vi "PIDController_Calculate_PV.vi"(10 "PV":dbl, 11 "in PID_CONTROLLER":T1={"Kp"=0.0, "Ki"=0.0, "Kd"=0.0, "Period"=0.0, "Max_Integral"=0.0, "Min_Integral"=0.0, "Max_Input"=0.0, "Min_Input"=0.0, "Continuous"=FALSE, "PositionError"=0.0, "VelocityError"=0.0, "PrevError"=0.0, "Total_Integral"=0.0, "PositionTolerance"=0.0, "VelocityTolerance"=0.0, "SetPoint"=0.0, "Kf"=0.0, "Prev_Deriv"=0.0, "Prev_Deriv 2"=0.0, "DerivativeFilter"=FALSE, "Min_Output"=-9.99e+35, "Max_Output"=9.9e+35, "Prev_F_P"=0.0, "Prev_F_P_2"=0.0, "AntiWindupActive"=FALSE, "Measurement"=0.0, "IntegralZone"=9.9e+30} {"IntegralZone" format="%16_6e"; "Measurement" format="%16_6e"; "Prev_F_P_2" format="%16_6e"; "Prev_F_P" format="%16_6e"; "Max_Output" format="%16_6e"; "Min_Output" format="%16_6e"; "Prev_Deriv 2" format="%16_6e"; "Prev_Deriv" format="%16_6e"; "Kf" format="%16_6e"; "SetPoint" format="%16_6e"; "VelocityTolerance" format="%16_6e"; "PositionTolerance" format="%16_6e"; "Total_Integral" format="%16_6e"; "PrevError" format="%16_6e"; "VelocityError" format="%16_6e"; "PositionError" format="%16_6e"; "Min_Input" format="%16_6e"; "Max_Input" format="%16_6e"; "Min_Integral" format="%16_6e"; "Max_Integral" format="%16_6e"; "Period" format="%16_6e"; "Kd" format="%16_6e"; "Ki" format="%16_6e"; "Kp" format="%16_6e"}) -> (1 "ControlOutput":dbl, 3 "out PID_CONTROLLER":T1={"Kp"=0.0, "Ki"=0.0, "Kd"=0.0, "Period"=0.0, "Max_Integral"=0.0, "Min_Integral"=0.0, "Max_Input"=0.0, "Min_Input"=0.0, "Continuous"=FALSE, "PositionError"=0.0, "VelocityError"=0.0, "PrevError"=0.0, "Total_Integral"=0.0, "PositionTolerance"=0.0, "VelocityTolerance"=0.0, "SetPoint"=0.0, "Kf"=0.0, "Prev_Deriv"=0.0, "Prev_Deriv 2"=0.0, "DerivativeFilter"=FALSE, "Min_Output"=-9.99e+35, "Max_Output"=9.9e+35, "Prev_F_P"=0.0, "Prev_F_P_2"=0.0, "AntiWindupActive"=FALSE, "Measurement"=0.0, "IntegralZone"=9.9e+30} {"IntegralZone" format="%16_6e"; "Measurement" format="%16_6e"; "Prev_F_P_2" format="%16_6e"; "Prev_F_P" format="%16_6e"; "Max_Output" format="%16_6e"; "Min_Output" format="%16_6e"; "Prev_Deriv 2" format="%16_6e"; "Prev_Deriv" format="%16_6e"; "Kf" format="%16_6e"; "SetPoint" format="%16_6e"; "VelocityTolerance" format="%16_6e"; "PositionTolerance" format="%16_6e"; "Total_Integral" format="%16_6e"; "PrevError" format="%16_6e"; "VelocityError" format="%16_6e"; "PositionError" format="%16_6e"; "Min_Input" format="%16_6e"; "Max_Input" format="%16_6e"; "Min_Integral" format="%16_6e"; "Max_Integral" format="%16_6e"; "Period" format="%16_6e"; "Kd" format="%16_6e"; "Ki" format="%16_6e"; "Kp" format="%16_6e"})   [LabVIEW 2019, in "Trajectory_Library.lvlib"]
doc: "Returns the next output of the PID controller. The saved setpoint (SP) in the PID_Controller data structure is used.\n \nInputs:\n - PID_Controller -- PID_Controller data cluster\n - PV-measurement -- The current measurement of the process variable. (PV)\n\nOutputs:\n - PID_Controller -- Updated PID_Controller data cluster\n - CO-ControlOutput -- Controller output (CO)"
uses:
  Trajectory_Library.lvlib
  TypeDef/PID_CONTROLLER.ctl
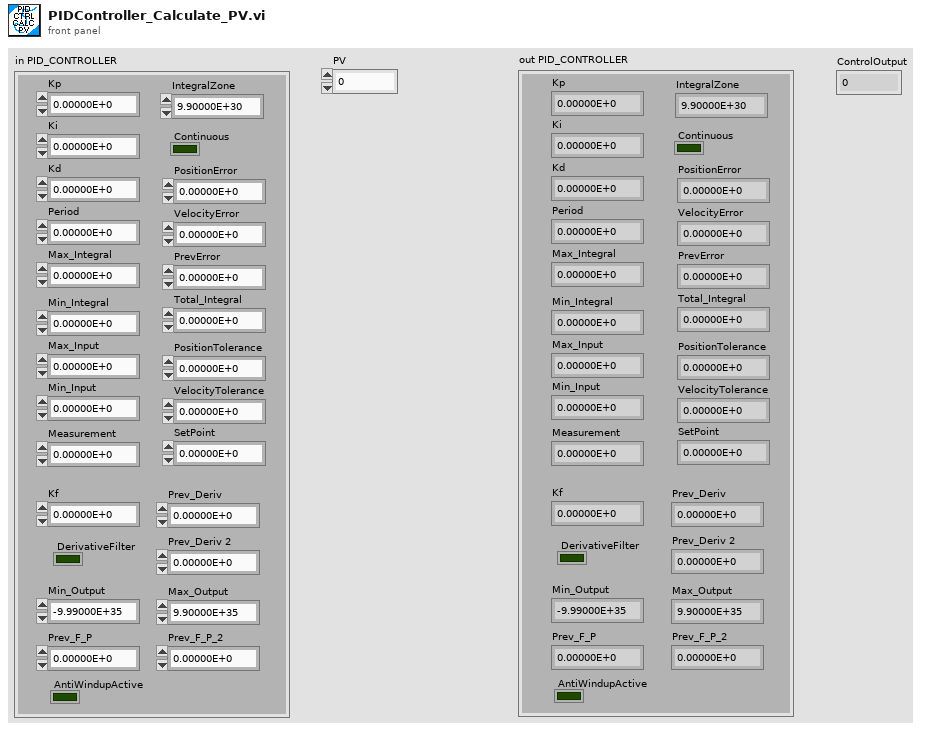
[diagram p1: front panel]
types:
  T1 = typedef "Trajectory_Library.lvlib/PID_CONTROLLER.ctl" = cluster{"Kp":dbl, "Ki":dbl, "Kd":dbl, "Period":dbl, "Max_Integral":dbl, "Min_Integral":dbl, "Max_Input":dbl, "Min_Input":dbl, "Continuous":bool, "PositionError":dbl, "VelocityError":dbl, "PrevError":dbl, "Total_Integral":dbl, "PositionTolerance":dbl, "VelocityTolerance":dbl, "SetPoint":dbl, "Kf":dbl, "Prev_Deriv":dbl, "Prev_Deriv 2":dbl, "DerivativeFilter":bool, "Min_Output":dbl, "Max_Output":dbl, "Prev_F_P":dbl, "Prev_F_P_2":dbl, "AntiWindupActive":bool, "Measurement":dbl, "IntegralZone":dbl}
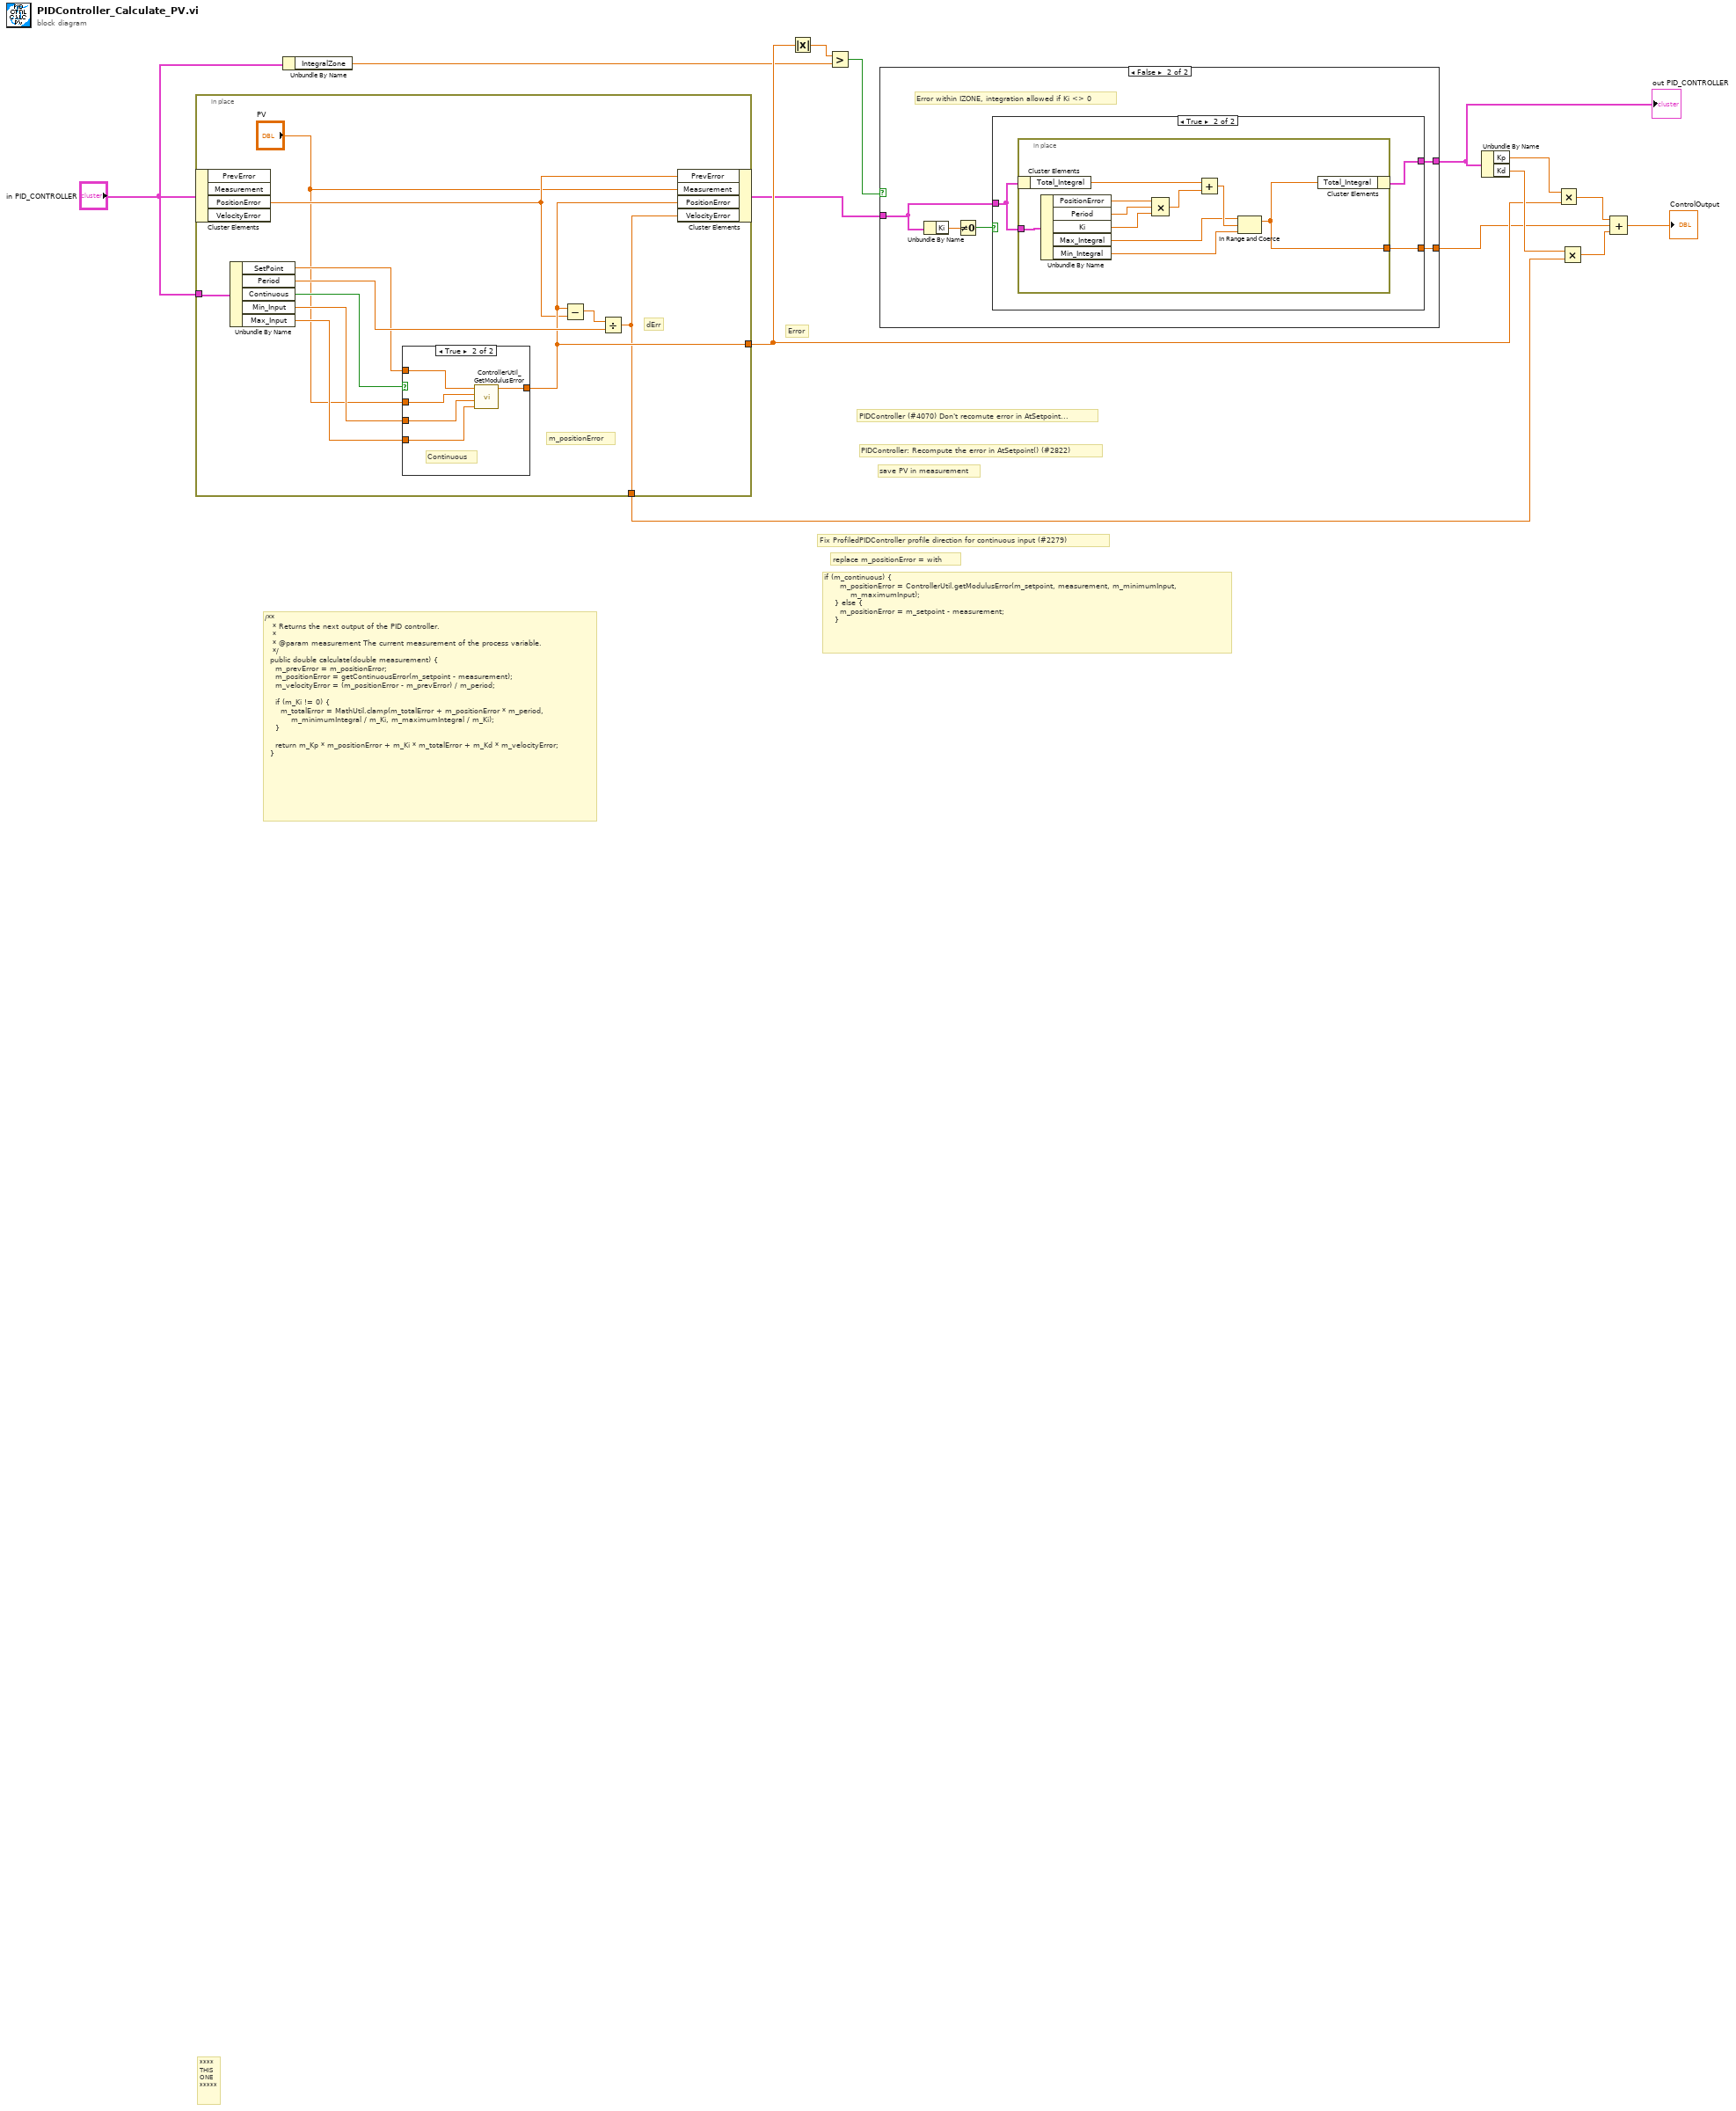
[diagram p0: block diagram]
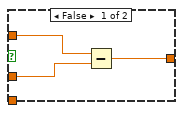
[diagram p2: hidden frame]
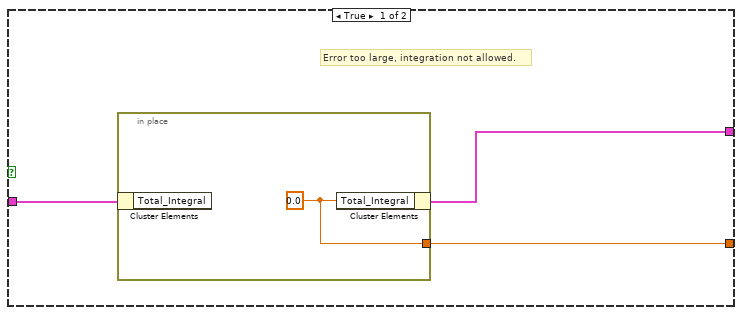
[diagram p3: hidden frame]
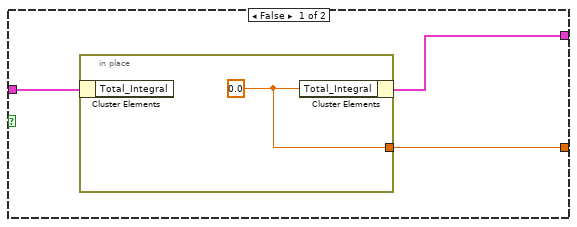
[diagram p4: hidden frame]
diagram:
  # "Error"
  # "PIDController (#4070) Don't recomute error in AtSetpoint..."
  # "save PV in measurement"
  # "PIDController: Recompute the error in AtSetpoint() (#2822)"
  # "Fix ProfiledPIDController profile direction for continuous input (#2279)"
  # "replace m_positionError = with"
  # "if (m_continuous) {\n      m_positionError = ControllerUtil.getModulusError(m_setpoint, measurement, m_minimumInput,\n          m_maximumInput);\n    } else {\n      m_positionError = m_setpoint - measurement;\n    }"
  # "/**\n   * Returns the next output of the PID controller.\n   *\n   * @param measurement The current measurement of the process variable.\n   */\n  public double calculate(double measurement) {\n    m_prevError = m_positionError;\n    m_positionError = getContinuousError(m_setpoint - measurement);\n    m_velocityError = (m_positionError - m_prevError) / m_period;\n\n    if (m_Ki != 0) {\n      m_totalError = MathUtil.clamp(m_totalError + m_positionError * m_period,\n          m_minimumIntegral / m_Ki, m_maximumIntegral / m_Ki);\n    }\n\n    return m_Kp * m_positionError + m_Ki * m_totalError + m_Kd * m_velocityError;\n  }"
  # "****\nTHIS\nONE\n*****"
  n1 = in-place {
    in-place-border: [w17] -> w8
    in-place-border: "in PID_CONTROLLER" -> [w19]
    in-place-border: [w18] -> w7
    # "dErr"
    # "m_positionError"
    n2 = in-place-cluster #1("in PID_CONTROLLER") -> ("PositionError"=w16:dbl)  [unwired: 3 out]
    n3 = Unbundle By Name(w19) -> ("SetPoint"=w22:dbl, "Period"=w24:dbl, "Continuous"=w23:bool, "Min_Input"=w21:dbl, "Max_Input"=w20:dbl)
    n4 = case shown="True" w23 {
      tunnel: w22 -> [w28 w33]
      tunnel: "PV" -> [w27 w32]
      tunnel: [w26 w29] -> w18
      tunnel: w21 -> [_ w31]
      tunnel: w20 -> [_ w30]
      frame False {
        n5 = Subtract(x=w28, y=w27) -> (x-y=w26:dbl)
      }
      frame True {
        # "Continuous"
        n6 = call "ControllerUtil_GetModulusError.vi"("Maximum_Input"=w30, "Minimum_Input"=w31, "Measurerment(PV)"=w32, "Reference(SP)"=w33) -> ("Error"=w29:dbl)  [unwired: 7 in]
      }
    }
    n7 = Subtract(x=w18, y=w16) -> (x-y=w25:dbl)
    n8 = Divide(x=w25, y=w24) -> (x/y=w17:dbl)
    n9 = in-place-cluster #1("PrevError"=w16, "Measurement"="PV", "PositionError"=w18, "VelocityError"=w17) -> (w4:T1)
  }
  n10 = Unbundle By Name("in PID_CONTROLLER") -> ("IntegralZone"=w2:dbl)
  n11 = Absolute Value(x=w7) -> (abs(x)=w6:dbl)
  n12 = Greater?(x=w6, y=w2) -> (0:w5:bool)
  n13 = case shown="False" w5 {
    tunnel: [w35 w40] -> w10
    tunnel: [w34 w39] -> w1
    tunnel: w4 -> [w36 w38]
    frame True {
      # "Error too large, integration not allowed."
      n14 = in-place {
        in-place-border: [w37] -> w34
        w37 = 0.0 ("TotalError")
        n15 = in-place-cluster #2(w36) -> ()  [unwired: 1 out]
        n16 = in-place-cluster #2("Total_Integral"=w37) -> (w35:T1)
      }
    }
    frame False {
      # "Error within IZONE, integration allowed if Ki <> 0"
      n17 = Unbundle By Name(w38) -> ("Ki"=w42:dbl)
      n18 = Not Equal To 0?(x=w42) -> (x != 0?=w41:bool)
      n19 = case shown="True" w41 {
        tunnel: w38 -> [w44 w48]
        tunnel: [w43 w47] -> w40
        tunnel: [w45 w49] -> w39
        frame False {
          n20 = in-place {
            in-place-border: [w46] -> w45
            w46 = 0.0 ("TotalError")
            n21 = in-place-cluster #3(w44) -> ()  [unwired: 1 out]
            n22 = in-place-cluster #3("Total_Integral"=w46) -> (w43:T1)
          }
        }
        frame True {
          n23 = in-place {
            in-place-border: w48 -> [w56]
            in-place-border: [w54] -> w49
            n24 = in-place-cluster #4(w48) -> ("Total_Integral"=w55:dbl)
            n25 = Unbundle By Name(w56) -> ("PositionError"=w59:dbl, "Period"=w58:dbl, "Ki"=w53:dbl, "Max_Integral"=w51:dbl, "Min_Integral"=w50:dbl)
            n26 = Compound Arithmetic op=MULTIPLY(w59, w58, w53) -> (w52:dbl)
            n27 = Add(x=w55, y=w52) -> (x+y=w57:dbl)
            n28 = In Range and Coerce(upper limit=w51, x=w57, lower limit=w50) -> (coerced(x)=w54:dbl)  [unwired: 1 out]
            n29 = in-place-cluster #4("Total_Integral"=w54) -> (w47:T1)
          }
        }
      }
    }
  }
  "out PID_CONTROLLER" <- w10
  n30 = Unbundle By Name(w10) -> ("Kp"=w12:dbl, "Kd"=w11:dbl)
  n31 = Multiply(x=w12, y=w7) -> (x*y=w14:dbl)
  n32 = Multiply(x=w11, y=w8) -> (x*y=w13:dbl)
  n33 = Compound Arithmetic op=ADD(w14, w1, w13) -> (→"ControlOutput":dbl)
